vi "Dynamic Shared Variable and Alarm Example (Prototype).vi"() -> ()   [LabVIEW 2021, in "Dynamic Shared Variables.lvlib"]
doc: "A prototype of the alarm code and UI display."
uses:
  Dynamic Shared Variables.lvlib
  Tag VIs/Tag FGV Operation Enum.ctl
  Alarm History.vi
  <vilib>/lvdsc/NI_DSC.lvlib
  Alarm Cluster.ctl
  Alarm Cluster (UI).ctl
panel:
  out "Alarm Event Time":timestamp
  out "output cluster":T1
  in  "Set Alarm Config":bool
  out "error out 2":errorcluster
  in  "my bool":bool
  in  "Alarm History Button":bool
  in  "UI Alarms":T2[](array[typedef])
  in  "TT1 Alarms":T3(array[cluster])=[{"enable? (F)"=TRUE, "name"="TT1:HiHi", "alarm type"=enum."HI_HI", "level/change"=80.0, "deadband/time"=1.0, "priority"=100, "ack type"=enum."Each Occurrence", "area"="", "description"="", "log? (T)"=TRUE}, {"enable? (F)"=TRUE, "name"="TT1:Hi", "alarm type"=enum."HI", "level/change"=70.0, "deadband/time"=1.0, "priority"=1, "ack type"=enum."Each Occurrence", "area"="", "description"="", "log? (T)"=TRUE}, {"enable? (F)"=TRUE, "name"="TT1:Lo", "alarm type"=enum."LO", "level/change"=30.0, "deadband/time"=1.0, "priority"=1, "ack type"=enum."Each Occurrence", "area"="", "description"="", "log? (T)"=TRUE}, {"enable? (F)"=TRUE, "name"="TT1:LoLo", "alarm type"=enum."LO_LO", "level/change"=20.0, "deadband/time"=1.0, "priority"=100, "ack type"=enum."Each Occurrence", "area"="", "description"="", "log? (T)"=TRUE}]
  in  "Alarm Model":T4[](array[typedef])=[{"Color Box"=16774466, "Name"="Temp:Hi", "Ack"=FALSE, "Alarm"={"alarm URL"="", "set time"=timestamp(3634824639.8324924 s since 1904-01-01), "set user"="(Nobody)", "ack time"=timestamp(-9223372036854775808 s since 1904-01-01), "ack user"="", "clear time"=timestamp(-9223372036854775808 s since 1904-01-01), "clear user"="", "setpoint"=30.0, "value"=22.498404260798484, "priority"=1, "alarm area"="", "alarm description"="", "ack comment"="", "event?"=FALSE, "Refnum"=216172782113783883}}, {"Color Box"=16711767, "Name"="Temp:HiHi", "Ack"=FALSE, "Alarm"={"alarm URL"="", "set time"=timestamp(3634824639.8324924 s since 1904-01-01), "set user"="(Nobody)", "ack time"=timestamp(-9223372036854775808 s since 1904-01-01), "ack user"="", "clear time"=timestamp(-9223372036854775808 s since 1904-01-01), "clear user"="", "setpoint"=30.0, "value"=22.498404260798484, "priority"=1, "alarm area"="", "alarm description"="", "ack comment"="", "event?"=FALSE, "Refnum"=216172782113783883}}, {"Color Box"=16774466, "Name"="Temp:Lo", "Ack"=FALSE, "Alarm"={"alarm URL"="", "set time"=timestamp(3634824639.8324924 s since 1904-01-01), "set user"="(Nobody)", "ack time"=timestamp(-9223372036854775808 s since 1904-01-01), "ack user"="", "clear time"=timestamp(-9223372036854775808 s since 1904-01-01), "clear user"="", "setpoint"=30.0, "value"=22.498404260798484, "priority"=1, "alarm area"="", "alarm description"="", "ack comment"="", "event?"=FALSE, "Refnum"=216172782113783883}}, {"Color Box"=16777216, "Name"="Temp:LoLo", "Ack"=FALSE, "Alarm"={"alarm URL"="", "set time"=timestamp(3634824639.8324924 s since 1904-01-01), "set user"="(Nobody)", "ack time"=timestamp(-9223372036854775808 s since 1904-01-01), "ack user"="", "clear time"=timestamp(-9223372036854775808 s since 1904-01-01), "clear user"="", "setpoint"=30.0, "value"=22.498404260798484, "priority"=1, "alarm area"="", "alarm description"="", "ack comment"="", "event?"=FALSE, "Refnum"=216172782113783883}}] {"Alarm"."value" format="%.2f"; "Alarm"."setpoint" format="%.2f"; "Alarm"."clear time" format="%<%X\n%x>T"; "Alarm"."ack time" format="%<%X\n%x>T"; "Alarm"."set time" format="%<%X\n%x>T"}
  in  "TT1 Value":dbl(knob)=51.86423922903216 scale=0.0..100.0
  out "error out":errorcluster
  in  "stop":bool
  out "alarms":T5(array[cluster])=[{"alarm URL"="\\\\Nate-VM-LV2018\\Pfizer FAST\\TT1.Alarms.Temp:Hi", "set time"=timestamp(3634823962.3858614 s since 1904-01-01), "set user"="(Nobody)", "ack time"=timestamp(3634823990.255854 s since 1904-01-01), "ack user"="(Nobody)", "clear time"=timestamp(-9223372036854775808 s since 1904-01-01), "clear user"="", "setpoint"=70.0, "value"=70.7018160134475, "priority"=1, "alarm area"="", "alarm description"="", "ack comment"="", "event?"=FALSE, "Refnum"=216172782113783876}, {"alarm URL"="\\\\Nate-VM-LV2018\\Pfizer FAST\\TT1.Alarms.Temp:HiHi", "set time"=timestamp(3634823996.2856817 s since 1904-01-01), "set user"="(Nobody)", "ack time"=timestamp(3634824000.485195 s since 1904-01-01), "ack user"="(Nobody)", "clear time"=timestamp(-9223372036854775808 s since 1904-01-01), "clear user"="", "setpoint"=80.0, "value"=80.9758251267968, "priority"=100, "alarm area"="", "alarm description"="", "ack comment"="", "event?"=FALSE, "Refnum"=216172782113783880}, {"alarm URL"="\\\\Nate-VM-LV2018\\Pfizer FAST\\TT2.Alarms.Temp:Lo", "set time"=timestamp(3634823976.465738 s since 1904-01-01), "set user"="(Nobody)", "ack time"=timestamp(-9223372036854775808 s since 1904-01-01), "ack user"="", "clear time"=timestamp(-9223372036854775808 s since 1904-01-01), "clear user"="", "setpoint"=50.0, "value"=48.61420716394651, "priority"=1, "alarm area"="", "alarm description"="", "ack comment"="", "event?"=FALSE, "Refnum"=216172782113783878}, {"alarm URL"="\\\\Nate-VM-LV2018\\Pfizer FAST\\TT2.Alarms.Temp:LoLo", "set time"=timestamp(3634823977.3064985 s since 1904-01-01), "set user"="(Nobody)", "ack time"=timestamp(-9223372036854775808 s since 1904-01-01), "ack user"="", "clear time"=timestamp(-9223372036854775808 s since 1904-01-01), "clear user"="", "setpoint"=30.0, "value"=29.741199723515926, "priority"=100, "alarm area"="", "alarm description"="", "ack comment"="", "event?"=FALSE, "Refnum"=216172782113783879}] {"value" format="%.2f"; "setpoint" format="%.2f"; "clear time" format="%<%X\n%x>T"; "ack time" format="%<%X\n%x>T"; "set time" format="%<%X\n%x>T"}
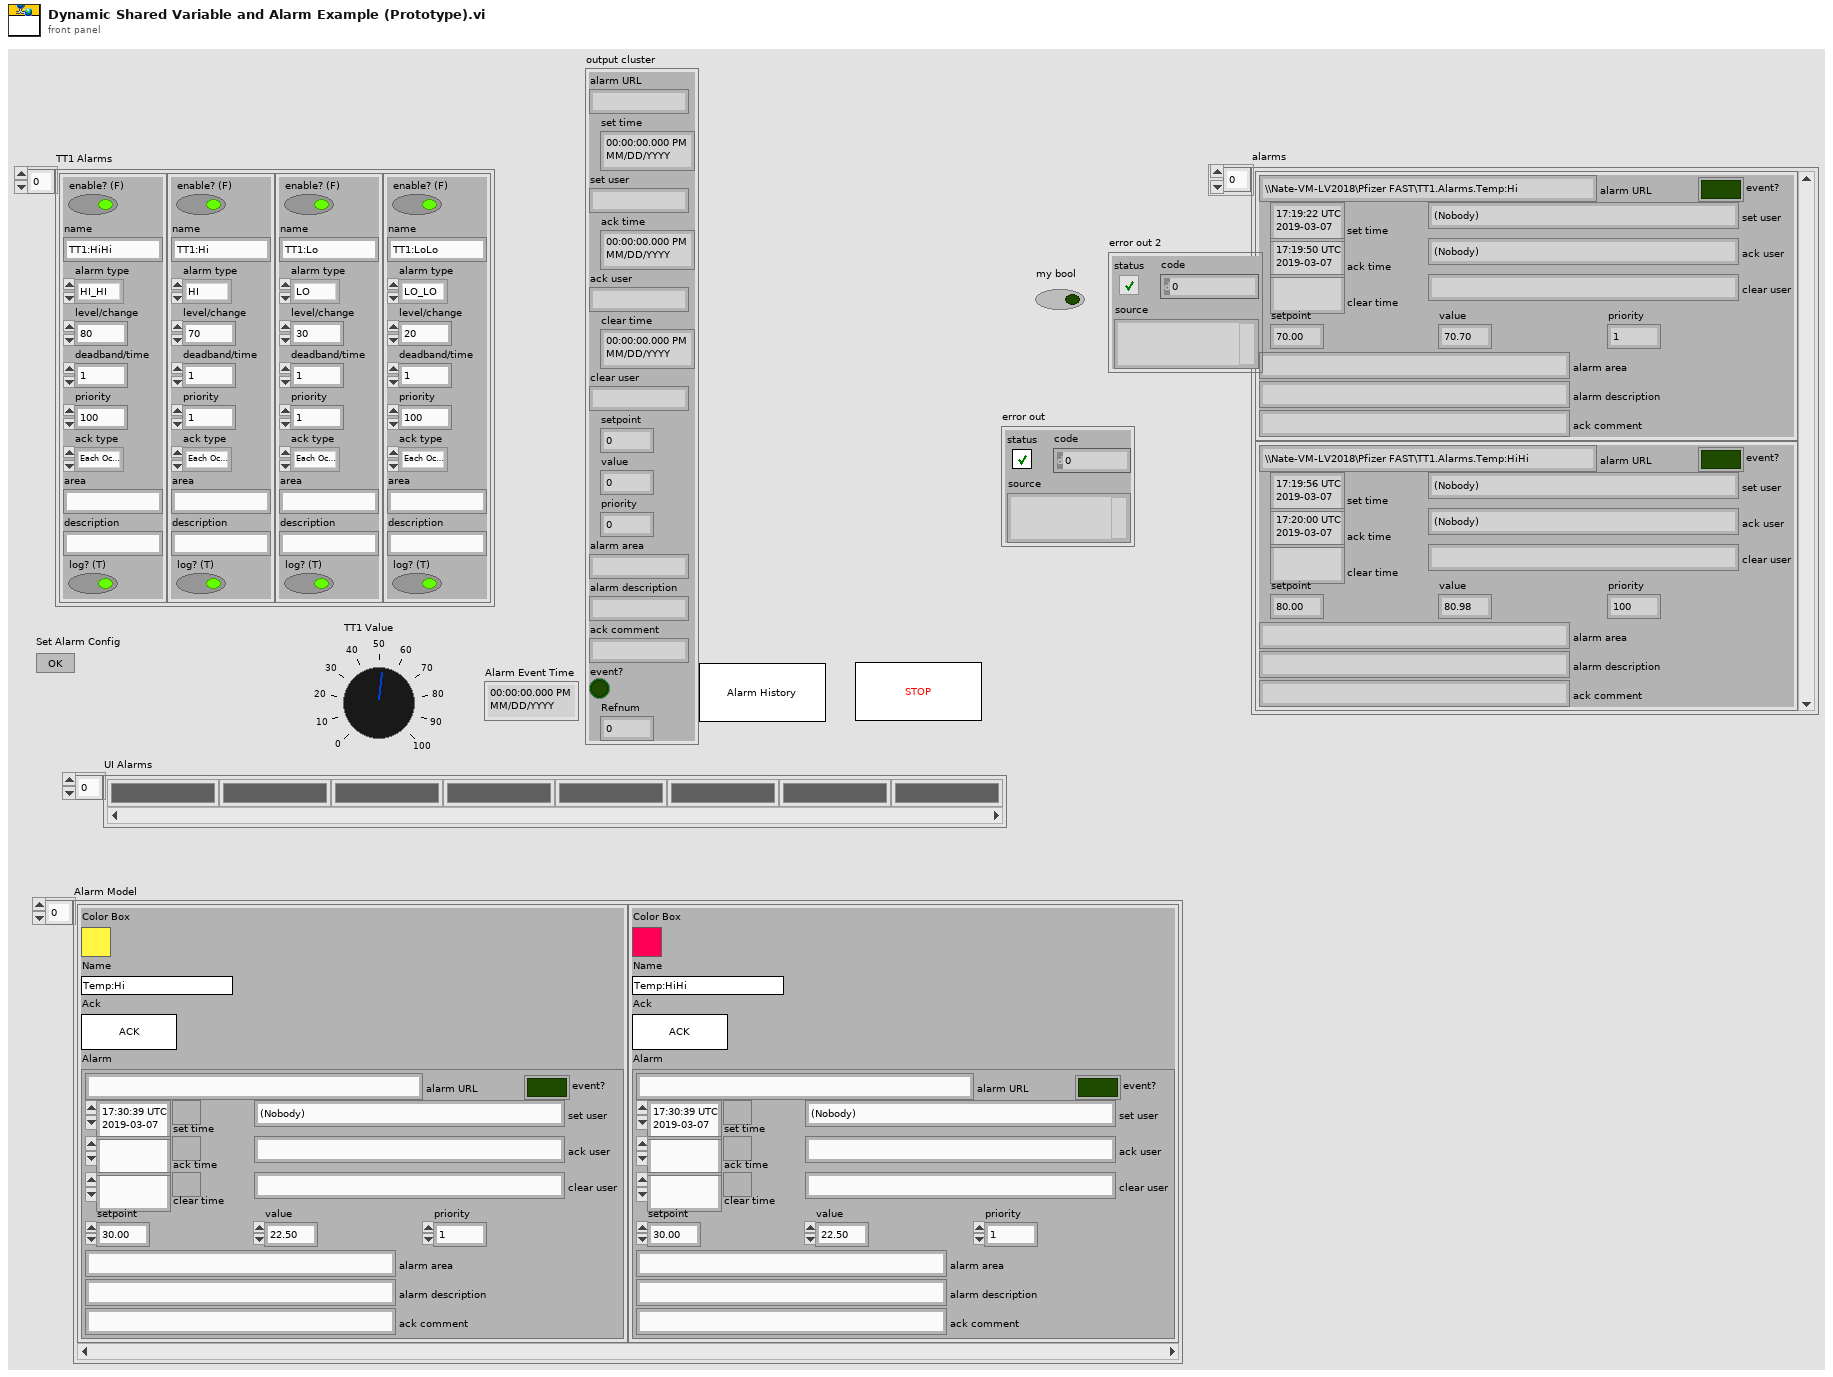
[diagram p1: front panel]
types:
  T1 = cluster{"alarm URL":string, "set time":timestamp, "set user":string, "ack time":timestamp, "ack user":string, "clear time":timestamp, "clear user":string, "setpoint":dbl, "value":dbl, "priority":u32, "alarm area":string, "alarm description":string, "ack comment":string, "event?":bool, "Refnum":u64}
  T2 = typedef "Dynamic Shared Variables.lvlib/Alarm Cluster (UI).ctl" = cluster{"Color Box":u32, "Name":string, "Ack":bool}
  T3 = cluster{"enable? (F)":bool, "name":string, "alarm type":enum16{"HI_HI", "HI", "LO", "LO_LO"}, "level/change":dbl, "deadband/time":dbl, "priority":u32, "ack type":enum16{"Auto", "User", "None", "Each Occurrence"}, "area":string, "description":string, "log? (T)":bool}[]
  T4 = typedef "Dynamic Shared Variables.lvlib/Alarm Cluster.ctl" = cluster{"Color Box":u32, "Name":string, "Ack":bool, "Alarm":cluster{"alarm URL":string, "set time":timestamp, "set user":string, "ack time":timestamp, "ack user":string, "clear time":timestamp, "clear user":string, "setpoint":dbl, "value":dbl, "priority":u32, "alarm area":string, "alarm description":string, "ack comment":string, "event?":bool, "Refnum":u64}}
  T5 = cluster{"alarm URL":string, "set time":timestamp, "set user":string, "ack time":timestamp, "ack user":string, "clear time":timestamp, "clear user":string, "setpoint":dbl, "value":dbl, "priority":u32, "alarm area":string, "alarm description":string, "ack comment":string, "event?":bool, "Refnum":u64}[]
  T6 = typedef "Tag FGV Operation Enum.ctl" = enum16{"Init", "Set Notification Queue", "Create Tag", "Commit", "Write Tag (Numeric)", "Write Tag (Boolean)", "Read All Tags", "Read One Tag", "Delete Tag Category", "Set Alarm Parameters (Numeric)", "Set Alarm Parameters (Boolean)", "Enable All Alarms", "Disable All Alarms", "Delete All Tags", "Read Alarms", "Ack Alarm", "Read Alarm Parameters (Numeric)", "Read Alarm Parameters (Boolean)"}
  T7 = enum32{"u32BitField", "bool", "double", "string", "int8", "uint8", "int16", "uint16", "int32", "uint32", "int64", "uint64", "single", "double waveform", "int16 waveform", "array of boolean", "array of int8", "array of uint8", "array of int16", "array of uint16", "array of int32", "array of uint32", "array of int64", "array of uint64", "array of single", "array of double", "array of double waveform", "array of int16 waveform", "array of string", "variant", "timestamp", "fixed point", "custom"}
  T8 = cluster{"Event Registration Refnum":refnum<event-registration>, "Stop Event Registration Refnum":refnum<event-registration>}
  T9 = enum32{"Invalid", "Standard", "Closed", "Hidden", "Minimized", "Maximized"}
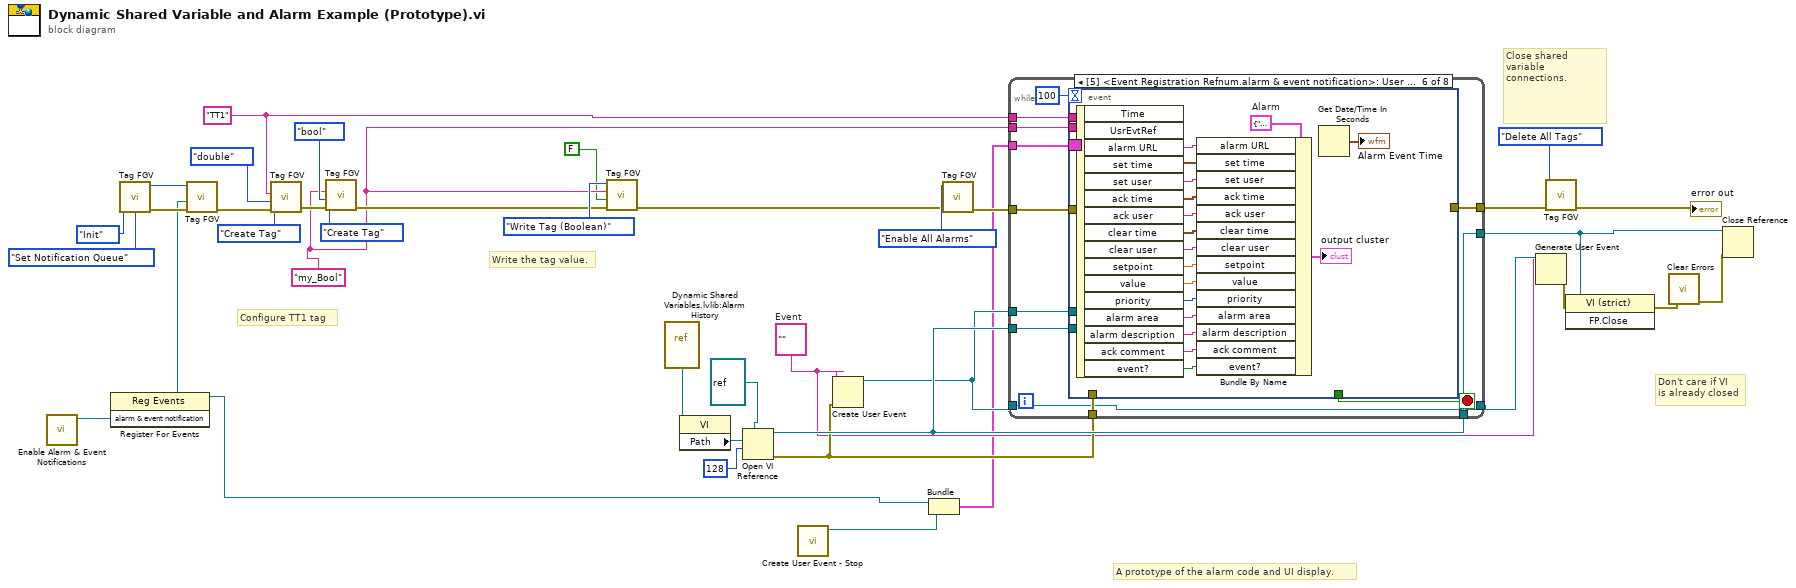
[diagram p0: block diagram]
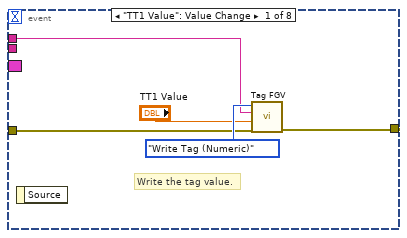
[diagram p2: hidden frame]
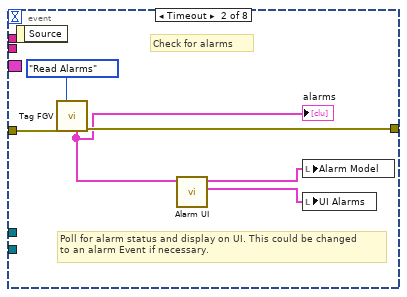
[diagram p3: hidden frame]
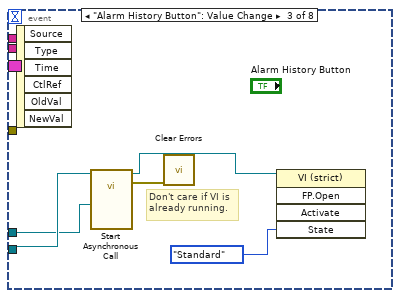
[diagram p4: hidden frame]
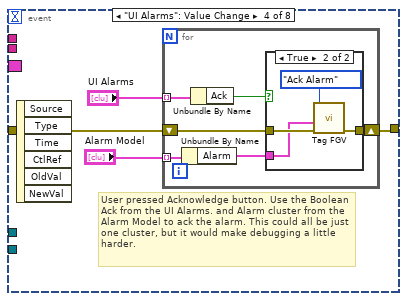
[diagram p5: hidden frame]
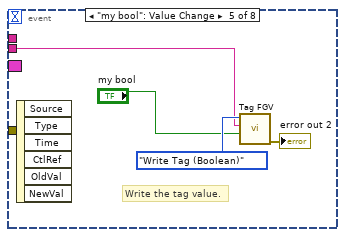
[diagram p7: hidden frame]
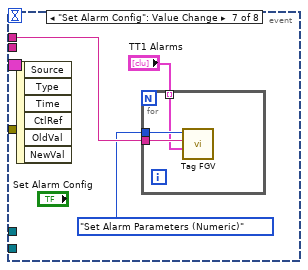
[diagram p8: hidden frame]
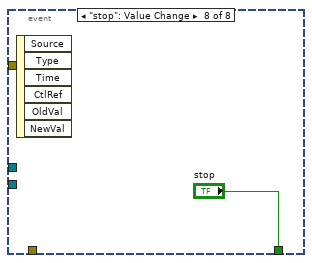
[diagram p9: hidden frame]
diagram:
  w10 = "my_Bool" ("Tag Name")
  w22 = ""  # Event
  w30 = "TT1" ("shared variable name")
  # "Write the tag value."
  # "Don't care if VI\nis already closed"
  # "Configure TT1 tag"
  # "A prototype of the alarm code and UI display."
  # "Close shared variable connections."
  n1 = call <vilib>:"Enable Alarm & Event Notifications.vi"() -> ("alarm & event notification"=w5:refnum<user-event>)  [unwired: 10 in, 1 out]
  n2 = register-events(w5) -> (reference out=w4:refnum<event-registration>)  [unwired: 2 in, 1 out]
  n3 = call "Tag FGV.vi"("Operation"=Tag_FGV_Operation_Enum."Init") -> ("error out"=w7:errorcluster)  [unwired: 5 in, 5 out]
  n4 = call "Tag FGV.vi"("error in (no error)"=w7, "Data"=w5, "Operation"=Tag_FGV_Operation_Enum."Set Notification Queue") -> ("error out"=w6:errorcluster)  [unwired: 3 in, 5 out]
  n5 = call "Tag FGV.vi"("error in (no error)"=w6, "Data"=T7."double" ("data type"), "Tag Name"=w30, "Operation"=Tag_FGV_Operation_Enum."Create Tag") -> ("error out"=w15:errorcluster)  [unwired: 2 in, 5 out]
  n6 = call "Tag FGV.vi"("error in (no error)"=w15, "Data"=T7."bool" ("data type"), "Tag Name"=w10, "Operation"=Tag_FGV_Operation_Enum."Create Tag") -> ("error out"=w11:errorcluster)  [unwired: 2 in, 5 out]
  n7 = call "Tag FGV.vi"("error in (no error)"=w11, "Data"=FALSE, "Tag Name"=w10, "Operation"=Tag_FGV_Operation_Enum."Write Tag (Boolean)") -> ("error out"=w1:errorcluster)  [unwired: 2 in, 5 out]
  n8 = vi-ref "Dynamic Shared Variables.lvlib:Alarm History.vi"() -> (w28:refnum<vi>)
  n9 = property class="VI"(reference=w28) -> ("Path"=w29:path)  [unwired: 1 in, 2 out]
  n10 = Open VI Reference(type specifier VI Refnum (for type only)=refnum<vi> refnum, vi path=w29, options=128) -> (vi reference=w26:refnum<vi>, error out=w25:errorcluster)  [unwired: 3 in]
  n11 = call "Create User Event - Stop.vi"() -> ("Stop Event Registration Refnum"=w2:refnum<event-registration>)  [unwired: 9 in, 2 out]
  n12 = Create User Event(user event datatype=w22, error in=w25) -> (user event=w23:refnum<user-event>)  [unwired: 1 out]
  n13 = Bundle("Event Registration Refnum"=w4, "Stop Event Registration Refnum"=w2) -> (w3:T8)  [unwired: 1 in]
  n14 = call "Tag FGV.vi"("error in (no error)"=w1, "Operation"=Tag_FGV_Operation_Enum."Enable All Alarms") -> ("error out"=w31:errorcluster)  [unwired: 4 in, 5 out]
  n15 = while {
    tunnel: w31 -> [w49]
    tunnel: [w47] -> w35
    tunnel: w30 -> [w45]
    tunnel: w25 -> [w44]
    tunnel: w26 -> [w43]
    tunnel: [w42] -> w21
    tunnel: w26 -> [w42]
    tunnel: w23 -> [w41]
    tunnel: [w40] -> w24
    tunnel: w23 -> [w40]
    tunnel: w10 -> [w39]
    tunnel: w3 -> [w38]
    stop <- w48 stop-if-true
    n16 = event shown="[5] <Event Registration Refnum.alarm & event notification>: User Event" {
      selector: w38 -> [_ _ _ _ _ _ _ _]
      dyn-events: _ -> [_ _ _ _ _ _ _ _]
      timeout: 100 -> [_ _ _ _ _ _ _ _]
      tunnel: w49 -> [w51 w58 _ w69 _ _ _ _]
      tunnel: [_ _ _ _ _ _ _ "stop"] -> w48
      tunnel: [w50 w59 _ w68 _ _ _ _] -> w47
      tunnel: w45 -> [w52 _ _ _ _ _ w104 _]
      tunnel: w44 -> [_ _ _ _ _ _ _ _]
      tunnel: w43 -> [_ _ w63 _ _ _ _ _]
      tunnel: w41 -> [_ _ w61 _ _ _ _ _]
      tunnel: w39 -> [_ _ _ _ w83 _ _ _]
      event "TT1 Value": Value Change {
        # "Write the tag value."
        n17 = event-data() -> ()  [unwired: 1 in, 1 out]
        n18 = call "Tag FGV.vi"("error in (no error)"=w51, "Data"="TT1 Value", "Tag Name"=w52, "Operation"=Tag_FGV_Operation_Enum."Write Tag (Numeric)") -> ("error out"=w50:errorcluster)  [unwired: 2 in, 5 out]
      }
      event Timeout {
        # "Poll for alarm status and display on UI. This could be changed\nto an alarm Event if necessary."
        # "Check for alarms"
        n19 = event-data() -> ()  [unwired: 1 in, 1 out]
        n20 = call "Tag FGV.vi"("error in (no error)"=w58, "Operation"=Tag_FGV_Operation_Enum."Read Alarms") -> ("error out"=w59:errorcluster, "alarms"=w55:T5)  [unwired: 4 in, 4 out]
        "alarms" <- w55
        n21 = call "Alarm UI.vi"("alarms"=w55) -> ("UI Alarms"=w56:T2[], "Alarm Model"=w57:T4[])  [unwired: 9 in]
        n22 = local write "Alarm Model"(w57) -> ()
        n23 = local write "UI Alarms"(w56) -> ()
      }
      event "Alarm History Button": Value Change {
        # "Don't care if VI is\nalready running."
        n24 = event-data() -> ()  [unwired: 1 in, 6 out]
        n25 = call-by-ref "Start Asynchronous Call"(reference=w63, "user event"=w61) -> (reference out=w64:refnum<vi>, error out=w62:errorcluster)  [unwired: 12 in]
        n26 = call <vilib>:"Clear Errors.vi"("error in (no error)"=w62) -> ()  [unwired: 5 in, 2 out]
        n27 = invoke class="VI (strict)" method="FP.Open"(reference=w64, "State"=T9."Standard") -> ()  [unwired: 3 in, 5 out]
      }
      event "UI Alarms": Value Change {
        # "User pressed Acknowledge button. Use the Boolean Ack from the UI Alarms. and Alarm cluster from the Alarm Model to ack the alarm. This could all be just one cluster, but it would make debugging a little harder."
        n28 = event-data() -> ()  [unwired: 1 in, 6 out]
        n29 = for {
          shift-right: [w74] -> w68
          shift-left: w69 -> [w75]
          tunnel: "UI Alarms" -> [w73] mode=indexing
          tunnel: "Alarm Model" -> [w71] mode=indexing
          n30 = Unbundle By Name(w71) -> ("Alarm"=w70:T1)
          n31 = Unbundle By Name(w73) -> ("Ack"=w72:bool)
          n32 = case shown="True" w72 {
            tunnel: w75 -> [w76 w80]
            tunnel: [w76 w79] -> w74
            tunnel: w70 -> [_ w77]
            frame False {
            }
            frame True {
              n33 = call "Tag FGV.vi"("error in (no error)"=w80, "Data"=w77, "Operation"=Tag_FGV_Operation_Enum."Ack Alarm") -> ("error out"=w79:errorcluster)  [unwired: 3 in, 5 out]
            }
          }
        }
      }
      event "my bool": Value Change {
        # "Write the tag value."
        n34 = event-data() -> ()  [unwired: 1 in, 6 out]
        n35 = call "Tag FGV.vi"("Data"="my bool", "Tag Name"=w83, "Operation"=Tag_FGV_Operation_Enum."Write Tag (Boolean)") -> ("error out"=→"error out 2":errorcluster)  [unwired: 3 in, 5 out]
      }
      event User Event {
        w101 = T1 {"alarm URL"="", "set time"=timestamp(0 s since 1904-01-01), "set user"="", "ack time"=timestamp(0 s since 1904-01-01), "ack user"="", "clear time"=timestamp(0 s since 1904-01-01), "clear user"="", "setpoint"=0.0, "value"=0.0, "priority"=0, "alarm area"="", "alarm description"="", "ack comment"="", "event?"=FALSE, "Refnum"=0}  # Alarm
        n36 = event-data() -> ("alarm URL"=w100:string, "set time"=w99:timestamp, "set user"=w98:string, "ack time"=w97:timestamp, "ack user"=w96:string, "clear time"=w95:timestamp, "clear user"=w94:string, "setpoint"=w93:dbl, "value"=w92:dbl, "priority"=w91:u32, "alarm area"=w90:string, "alarm description"=w89:string, "ack comment"=w87:string, "event?"=w88:bool)  [unwired: 1 in, 2 out]
        n37 = Bundle By Name(cluster=w101, "alarm URL"=w100, "set time"=w99, "set user"=w98, "ack time"=w97, "ack user"=w96, "clear time"=w95, "clear user"=w94, "setpoint"=w93, "value"=w92, "priority"=w91, "alarm area"=w90, "alarm description"=w89, "ack comment"=w87, "event?"=w88) -> (→"output cluster":T1)
        n38 = Get Date/Time In Seconds() -> (seconds since 1Jan1904=→"Alarm Event Time":timestamp)
      }
      event "Set Alarm Config": Value Change {
        n39 = event-data() -> ()  [unwired: 1 in, 6 out]
        n40 = for {
          tunnel: Tag_FGV_Operation_Enum."Set Alarm Parameters (Numeric)" ("Operation") -> [w107]
          tunnel: w104 -> [w106]
          tunnel: "TT1 Alarms" -> [w105] mode=indexing
          n41 = call "Tag FGV.vi"("Data"=w105, "Tag Name"=w106, "Operation"=w107) -> ()  [unwired: 3 in, 6 out]
        }
      }
      event "stop": Value Change {
        n42 = event-data() -> ()  [unwired: 1 in, 6 out]
      }
    }
  }
  n43 = Generate User Event(user event=w24, event data cluster=w22) -> (error out=w20:errorcluster)  [unwired: 2 in, 1 out]
  n44 = call "Tag FGV.vi"("error in (no error)"=w35, "Operation"=Tag_FGV_Operation_Enum."Delete All Tags") -> ("error out"=→"error out":errorcluster)  [unwired: 4 in, 5 out]
  n45 = invoke class="VI (strict)" method="FP.Close"(reference=w21, error in=w20) -> (error out=w19:errorcluster)  [unwired: 1 in, 2 out]
  n46 = call <vilib>:"Clear Errors.vi"("error in (no error)"=w19) -> ("error out"=w18:errorcluster)  [unwired: 5 in, 1 out]
  n47 = Close Reference(reference=w21, error in (no error)=w18) -> ()  [unwired: 1 out]
